vi "Consulta bd v03.vi"(8 "error in (no error)":errorcluster, 11 "Database":T4) -> (0 "error out":errorcluster)   [LabVIEW 2017]
uses:
  <vilib>/addons/database/Connection.llb/Conn ObjectReference.ctl
  <vilib>/GPower/Array/Library/RemDup/RemDup_Str.vi
  <vilib>/GPower/Array/Library/RemDup/RemDup_Var.vi
  <vilib>/NI/AMC/Update Message Routing Info.vi
  <vilib>/NI/AMC/Create Multiple Messages.vi
  <vilib>/NI/AMC/Read Termination Message.vi
  <vilib>/NI/AMC/Create Single Message.vi
  <vilib>/NI/AMC/Send Message.vi
  <vilib>/NI/AMC/Globals.vi
  <userlib>/_OpenG.lib/array/array.llb/Sort 1D Array (String)__ogtk.vi
  <vilib>/addons/database/_DB Variant To Data/Database Variant To Data.xnode
  <vilib>/addons/database/NI_Database_API.lvlib
  <vilib>/NI/AMC/AMC.lvlib
  <vilib>/GPower/Array/GPArray.lvlib
panel:
  in  "System Tab":T1(tab)
  out "Picture":picture
  out "Horas por trabajador":T2(array[cluster])
  out "Horas totales (hh:mm)":string
  out "1D Array":T3(array[cluster])
  in  "Proyectos":string(combo)
  in  "Time Stamp Array":timestamp[](array[timestamp])
  in  "Salir":bool
  in  "Consultar":bool
  in  "Fecha de finalización":timestamp format="%<%.0X %x>T"
  in  "Fecha de inicio":timestamp format="%<%.0X %x>T"
  # "Consulta Base de Datos"
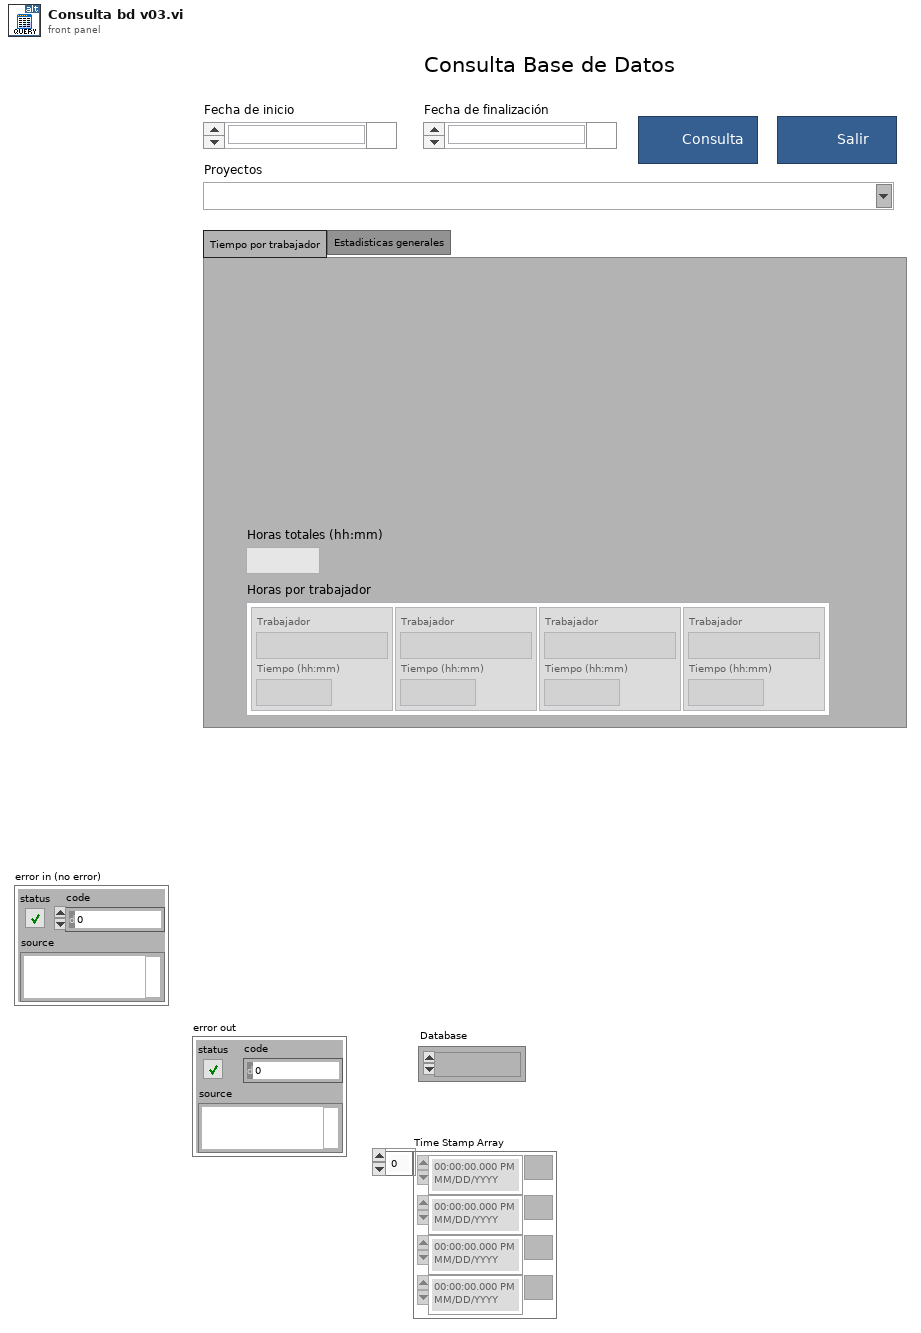
[diagram p1: front panel]
types:
  T1 = enum32{"Tiempo por trabajador", "Estadisticas generales"}
  T2 = cluster{"Trabajador":string, "Tiempo (hh:mm) ":string}[]
  T3 = cluster{"Trabajador":string, "Tarea":string, "Inicio":string, "Fin":string, "Duracion":dbl}[]
  T4 = typedef "NI_Database_API.lvlib/Conn ObjectReference.ctl" = refnum<k1>
  T5 = typedef "AMC.lvlib/Message Queue.ctl" = refnum<queue>
  T6 = cluster{"Trabajador":string, "Tarea":string, "Inicio":string, "Fin":string, "Duracion":i32}[]
  T7 = typedef "LVBoundsTypeDef.ctl" = cluster{"Width":u32, "Height":u32}
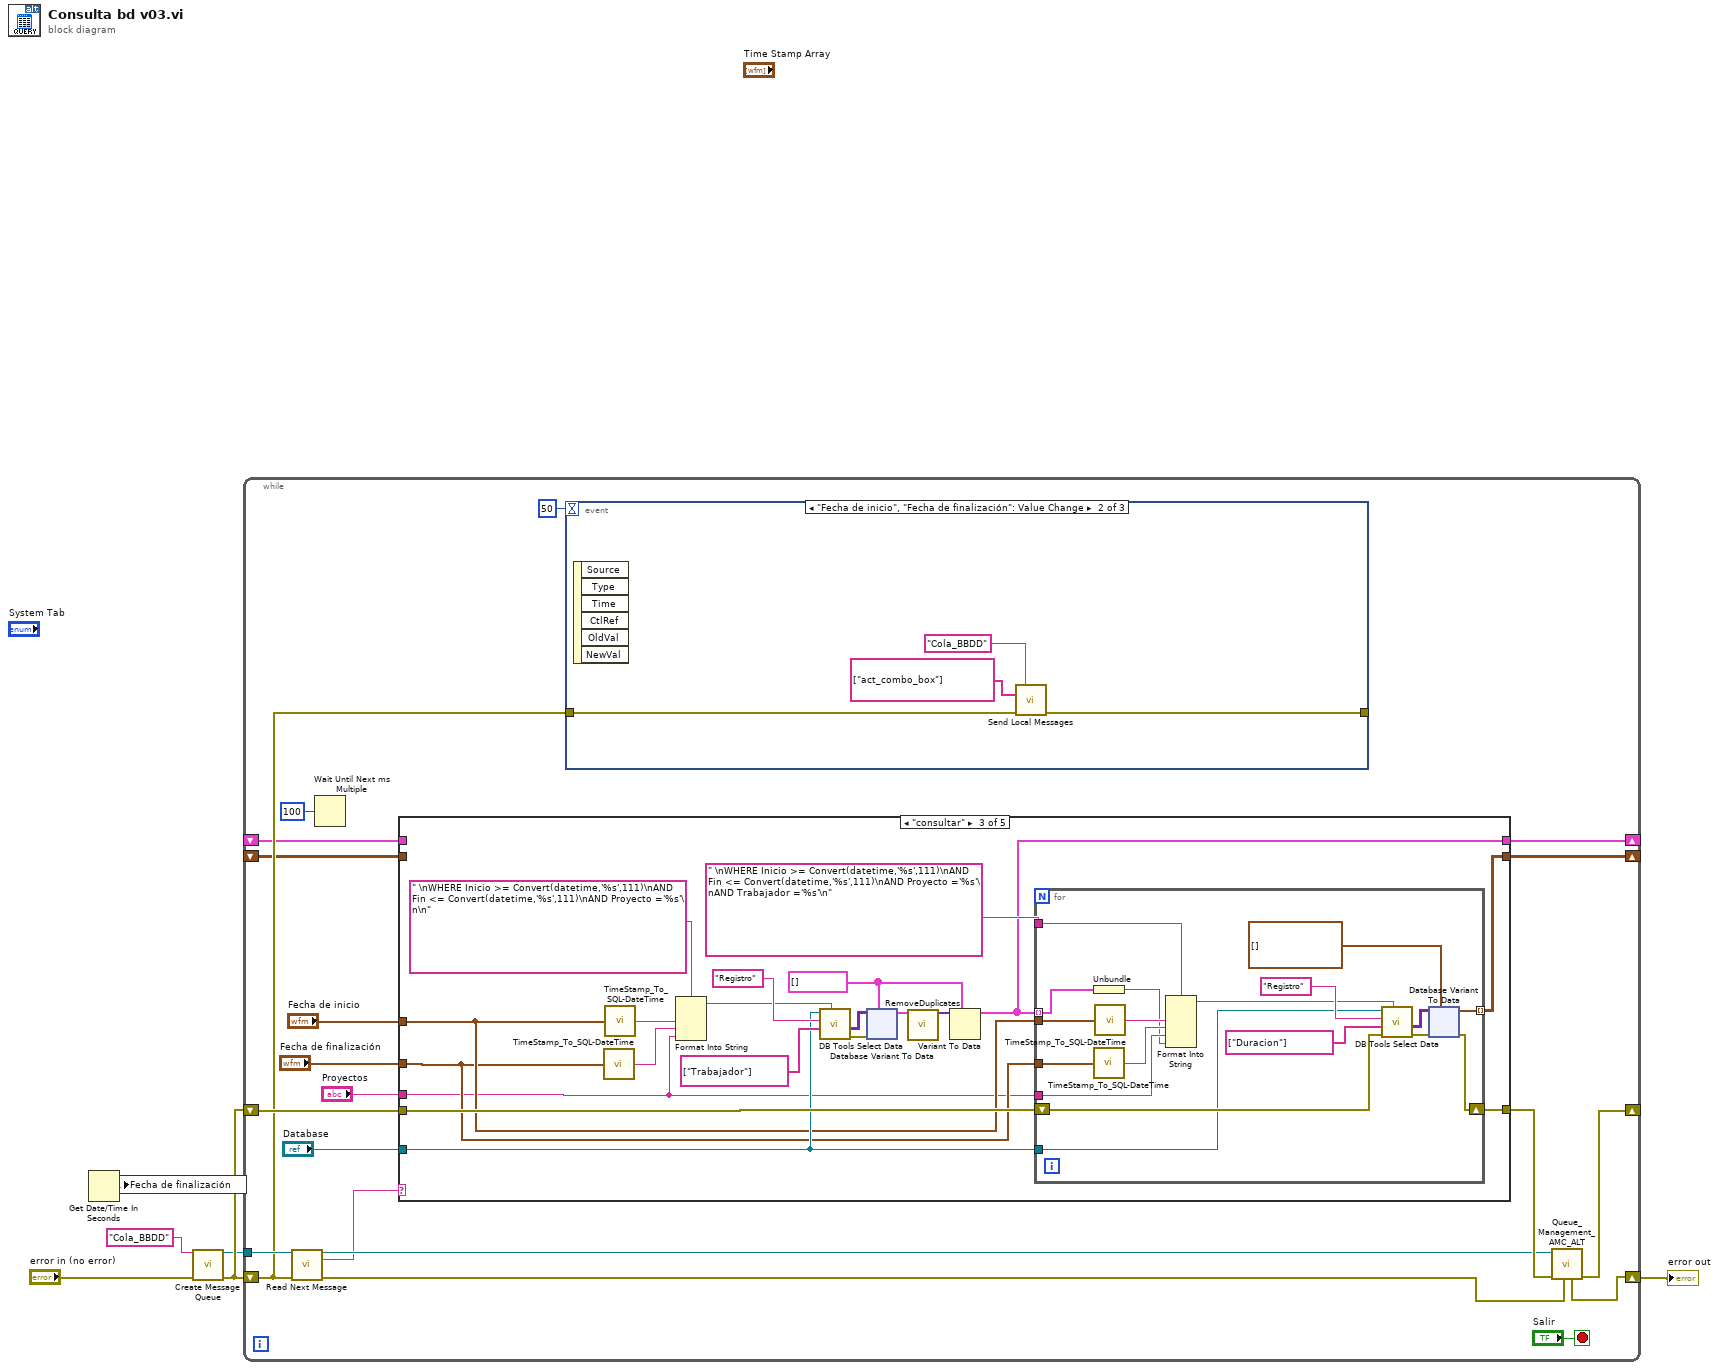
[diagram p0: block diagram]
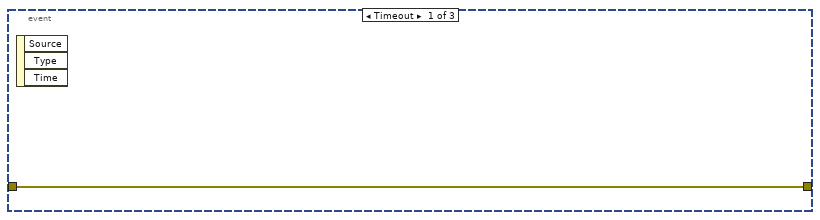
[diagram p2: hidden frame]
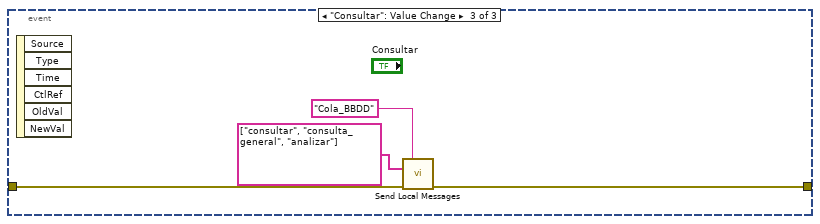
[diagram p3: hidden frame]
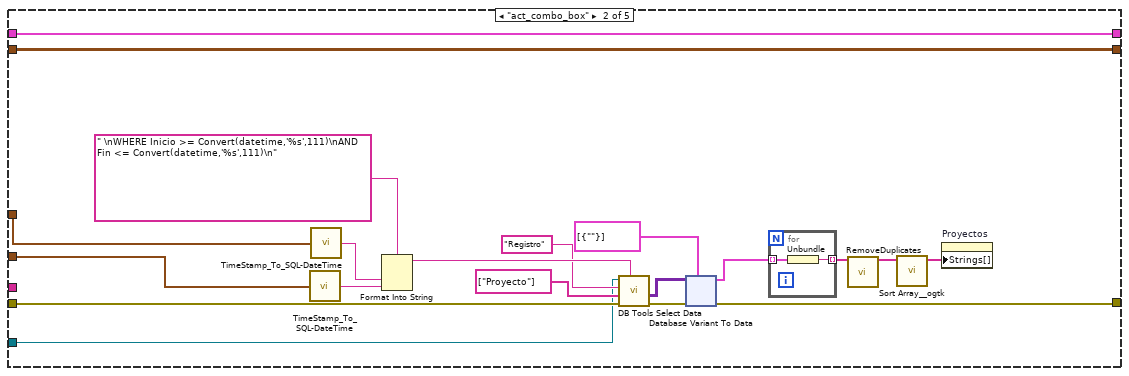
[diagram p5: hidden frame]
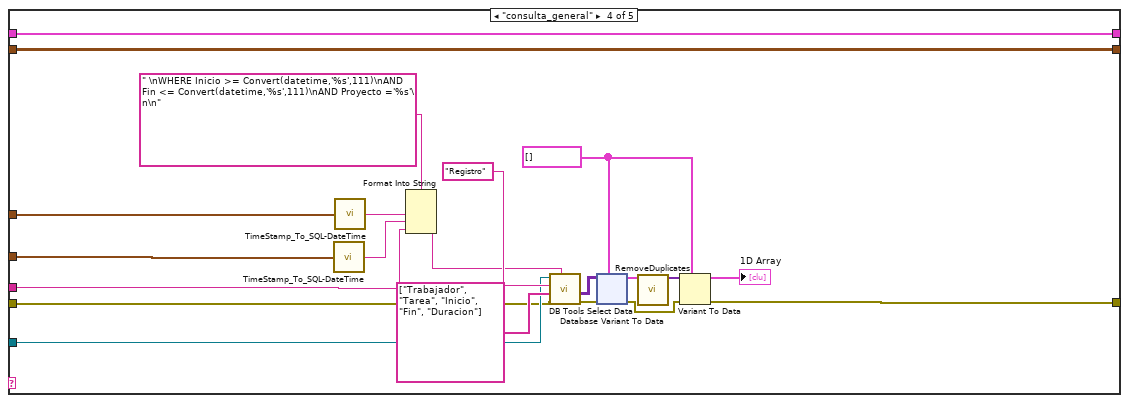
[diagram p6: hidden frame]
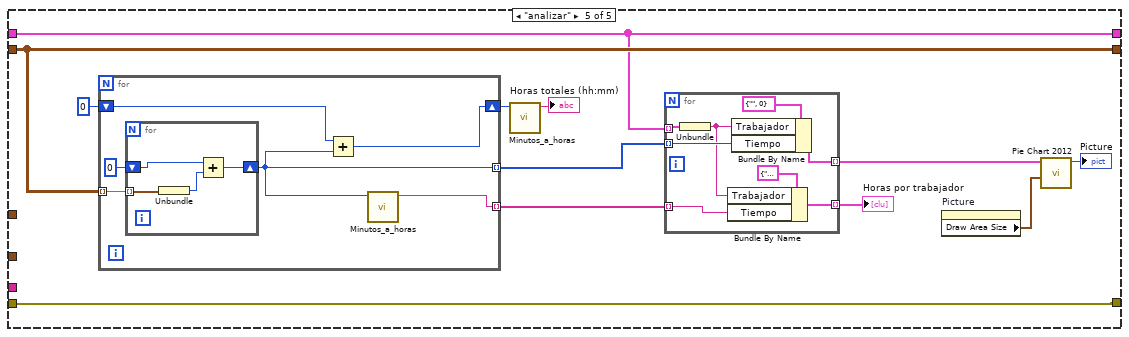
[diagram p7: hidden frame]
diagram:
  n1 = Get Date/Time In Seconds() -> (seconds since 1Jan1904=w3:timestamp)
  n2 = local write "Fecha de finalización"(w3) -> ()
  n3 = call <vilib>:"Create Message Queue.vi"("message queue name"="Cola_BBDD", "error in"="error in (no error)") -> ("message queue out"=w1:T5, "error out"=w2:errorcluster)  [unwired: 12 in]
  n4 = while {
    shift-right: [w18] -> w6
    shift-left: w2 -> [w13]
    tunnel: w1 -> [w20]
    shift-right: [w16] -> _
    shift-left: w2 -> [w21]
    shift-right: [w11] -> _
    shift-left: _ -> [w10]
    shift-right: [w9] -> _
    shift-left: _ -> [w8]
    stop <- "Salir" stop-if-true
    n5 = call <vilib>:"Read Next Message.vi"("message queue in"=w20, "error in"=w13) -> ("message queue out"=w15:T5, "message name"=w14:string, "error out"=w19:errorcluster)  [unwired: 6 in, 5 out]
    n6 = Wait Until Next ms Multiple(millisecond multiple=u32 100) -> ()  [unwired: 1 out]
    n7 = case shown="\"consultar\"" w14 {
      tunnel: w21 -> [w38 w47 w120 w226 w419]
      tunnel: [w38 w44 w121 w224 w419] -> w17
      tunnel: "Fecha de inicio" -> [_ w46 w105 w230 _]
      tunnel: "Fecha de finalización" -> [_ w48 w104 w229 _]
      tunnel: "Database" -> [_ w45 w111 w235 _]
      tunnel: [w37 w43 w116 w227 w416] -> w11
      tunnel: w10 -> [w37 w43 _ w227 w416]
      tunnel: [w36 w42 w103 w223 w414] -> w9
      tunnel: w8 -> [w36 w42 _ w223 w414]
      tunnel: "Proyectos" -> [_ _ w102 w228 _]
      frame "", Default {
      }
      frame "act_combo_box" {
        n8 = call "TimeStamp_To_SQL-DateTime.vi"("time stamp"=w48) -> ("date/time string"=w55:string)
        n9 = call "TimeStamp_To_SQL-DateTime.vi"("time stamp"=w46) -> ("date/time string"=w56:string)
        n10 = Format Into String(format string=" \nWHERE Inicio >= Convert(datetime,'%s',111)\nAND Fin <= Convert(datetime,'%s',111)\n" ("condition"), w56, w55) -> (resulting string=w52:string)  [unwired: 2 in, 1 out]
        n11 = call <vilib>:"DB Tools Select Data.vi"("condition"=w52, "error in (no error)"=w47, "columns"=string[] ["Proyecto"], "table"="Registro", "connection reference"=w45) -> ("error out"=w53:errorcluster, "data"=w58:variant[][])  [unwired: 1 in, 1 out]
        n12 = xnode "Database Variant To Data"("database variant"=w58, "error in (no error)"=w53, "type"=cluster{string}[] [{""}] ("Waveform Graph")) -> ("data"=w50:cluster{string}[], "error out"=w44:errorcluster)
        n13 = for {
          tunnel: w50 -> [w101] mode=indexing
          tunnel: [w100] -> w41 mode=indexing
          n14 = Unbundle(w101) -> (w100:string)
        }
        n15 = call-poly <vilib>:"RemoveDuplicates.vi"("Array"=w41) -> ("Array Without Duplicates"=w40:string[])  [unwired: 12 in, 2 out]
        n16 = call-poly <userlib>:"Sort Array__ogtk.vi"("Array in"=w40) -> ("Sorted Array out"=w39:string[])  [unwired: 9 in, 1 out]
        n17 = property on="Proyectos" class="CmbBox"("Strings[]"=w39) -> ()  [unwired: 2 in, 2 out]
      }
      frame "consultar" {
        w107 = cluster{"Trabajador":string}[] []
        n18 = call "TimeStamp_To_SQL-DateTime.vi"("time stamp"=w104) -> ("date/time string"=w117:string)
        n19 = call "TimeStamp_To_SQL-DateTime.vi"("time stamp"=w105) -> ("date/time string"=w118:string)
        n20 = Format Into String(format string=" \nWHERE Inicio >= Convert(datetime,'%s',111)\nAND Fin <= Convert(datetime,'%s',111)\nAND Proyecto ='%s'\n\n" ("condition"), w118, w117, w102) -> (resulting string=w110:string)  [unwired: 2 in, 1 out]
        n21 = call <vilib>:"DB Tools Select Data.vi"("condition"=w110, "columns"=string[] ["Trabajador"], "table"="Registro", "connection reference"=w111) -> ("error out"=w113:errorcluster, "data"=w112:variant[][])  [unwired: 2 in, 1 out]
        n22 = xnode "Database Variant To Data"("database variant"=w112, "error in (no error)"=w113, "type"=w107) -> ("data"=w109:cluster{"Trabajador":string}[])  [unwired: 1 out]
        n23 = call-poly <vilib>:"RemoveDuplicates.vi"("Array"=w109) -> ("Array with duplicates removed"=w106:variant[])  [unwired: 12 in, 2 out]
        n24 = Variant To Data(type=w107, Variant=w106) -> (data=w103:cluster{"Trabajador":string}[])  [unwired: 1 in, 1 out]
        n25 = for {
          tunnel: [w173] -> w116 mode=indexing
          tunnel: w111 -> [w172]
          tunnel: " \nWHERE Inicio >= Convert(datetime,'%s',111)\nAND Fin <= Convert(datetime,'%s',111)\nAND Proyecto ='%s'\nAND Trabajador ='%s'\n" ("condition") -> [w169]
          tunnel: w102 -> [w168]
          shift-right: [w180] -> w121
          shift-left: w120 -> [w179]
          tunnel: w103 -> [w167] mode=indexing
          tunnel: w105 -> [w164]
          tunnel: w104 -> [w163]
          n26 = Unbundle(w167) -> ("Trabajador"=w166:string)
          n27 = call "TimeStamp_To_SQL-DateTime.vi"("time stamp"=w163) -> ("date/time string"=w171:string)
          n28 = call "TimeStamp_To_SQL-DateTime.vi"("time stamp"=w164) -> ("date/time string"=w170:string)
          n29 = Format Into String(format string=w169, w170, w171, w168, w166) -> (resulting string=w165:string)  [unwired: 2 in, 1 out]
          n30 = call <vilib>:"DB Tools Select Data.vi"("condition"=w165, "error in (no error)"=w179, "columns"=string[] ["Duracion"], "table"="Registro", "connection reference"=w172) -> ("error out"=w177:errorcluster, "data"=w178:variant[][])  [unwired: 1 in, 1 out]
          n31 = xnode "Database Variant To Data"("database variant"=w178, "error in (no error)"=w177, "type"=cluster{"Duracion":i32}[] []) -> ("data"=w173:cluster{"Duracion":i32}[], "error out"=w180:errorcluster)
        }
      }
      frame "consulta_general" {
        w232 = T6 []
        n32 = call "TimeStamp_To_SQL-DateTime.vi"("time stamp"=w229) -> ("date/time string"=w240:string)
        n33 = call "TimeStamp_To_SQL-DateTime.vi"("time stamp"=w230) -> ("date/time string"=w241:string)
        n34 = Format Into String(format string=" \nWHERE Inicio >= Convert(datetime,'%s',111)\nAND Fin <= Convert(datetime,'%s',111)\nAND Proyecto ='%s'\n\n" ("condition"), w241, w240, w228) -> (resulting string=w234:string)  [unwired: 2 in, 1 out]
        n35 = call <vilib>:"DB Tools Select Data.vi"("condition"=w234, "error in (no error)"=w226, "columns"=string[] ["Trabajador", "Tarea", "Inicio", "Fin", "Duracion"], "table"="Registro", "connection reference"=w235) -> ("error out"=w237:errorcluster, "data"=w236:variant[][])  [unwired: 1 in, 1 out]
        n36 = xnode "Database Variant To Data"("database variant"=w236, "error in (no error)"=w237, "type"=w232) -> ("data"=w233:T6, "error out"=w225:errorcluster)
        n37 = call-poly <vilib>:"RemoveDuplicates.vi"("Array"=w233) -> ("Array with duplicates removed"=w231:variant[])  [unwired: 12 in, 2 out]
        n38 = Variant To Data(error in=w225, type=w232, Variant=w231) -> (data=→"1D Array":T6, error out=w224:errorcluster)
      }
      frame "analizar" {
        n39 = for {
          tunnel: w416 -> [w433] mode=indexing
          tunnel: [w430] -> w415 mode=indexing
          tunnel: [w431] -> w412 mode=indexing
          shift-right: [w429] -> w409
          shift-left: 0 -> [w428]
          n40 = for {
            tunnel: w433 -> [w437] mode=indexing
            shift-right: [w434] -> w430
            shift-left: 0 ("Duracion") -> [w436]
            n41 = Unbundle(w437) -> ("Duracion"=w435:i32)
            n42 = Add(x=w436, y=w435) -> (x+y=w434:i32)
          }
          n43 = Add(x=w428, y=w430) -> (x+y=w429:i32)
          n44 = call "Minutos_a_horas.vi"("Duracion"=w430) -> ("String"=w431:string)  [unwired: 10 in]
        }
        n45 = call "Minutos_a_horas.vi"("Duracion"=w409) -> ("String"=→"Horas totales (hh:mm)":string)  [unwired: 10 in]
        n46 = for {
          tunnel: w414 -> [w426] mode=indexing
          tunnel: w415 -> [w425] mode=indexing
          tunnel: [w424] -> w413 mode=indexing
          tunnel: w412 -> [w420] mode=indexing
          tunnel: [w421] -> w411 mode=indexing
          n47 = Unbundle(w426) -> ("Trabajador"=w423:string)
          n48 = Bundle By Name(cluster=cluster{"Trabajador":string, "Tiempo":string} {"Trabajador"="", "Tiempo"=""}, "Trabajador"=w423, "Tiempo"=w420) -> (w421:cluster{"Trabajador":string, "Tiempo":string})
          n49 = Bundle By Name(cluster=cluster{"Trabajador":string, "Tiempo":i32} {"Trabajador"="", "Tiempo"=0}, "Trabajador"=w423, "Tiempo"=w425) -> (w424:cluster{"Trabajador":string, "Tiempo":i32})
        }
        "Horas por trabajador" <- w411
        n50 = property on="Picture" class="Pict"() -> ("Draw Area Size"=w417:T7)  [unwired: 2 in, 2 out]
        n51 = call "Pie Chart 2012.vi"("Draw Area Size"=w417, "Array"=w413) -> ("Picture"=→"Picture":picture)  [unwired: 9 in]
      }
    }
    n52 = event shown="[1] \"Fecha de inicio\", \"Fecha de finalización\": Value Change" {
      selector: _ -> [_ _ _]
      dyn-events: _ -> [_ _ _]
      timeout: 50 -> [_ _ _]
      tunnel: w13 -> [w27 w29 w33]
      tunnel: [w27 w28 w32] -> _
      event Timeout {
        n53 = event-data() -> ()  [unwired: 1 in, 3 out]
      }
      event "Fecha de inicio", "Fecha de finalización": Value Change {
        n54 = event-data() -> ()  [unwired: 1 in, 6 out]
        n55 = call <vilib>:"Send Local Messages.vi"("receiver process (\"\" - local)"="Cola_BBDD" ("receiver process (\"\" - local)"), "message names"=string[] ["act_combo_box"] ("message name"), "error in"=w29) -> ("error out"=w28:errorcluster)  [unwired: 10 in, 2 out]
      }
      event "Consultar": Value Change {
        n56 = event-data() -> ()  [unwired: 1 in, 6 out]
        n57 = call <vilib>:"Send Local Messages.vi"("receiver process (\"\" - local)"="Cola_BBDD" ("receiver process (\"\" - local)"), "message names"=string[] ["consultar", "consulta_general", "analizar"] ("message name"), "error in"=w33) -> ("error out"=w32:errorcluster)  [unwired: 10 in, 2 out]
      }
    }
    n58 = call "Queue_Management_AMC_ALT.vi"("queue error in"=w19, "system error in"=w17, "message queue in"=w15) -> ("system error out"=w16:errorcluster, "queue error out"=w18:errorcluster)  [unwired: 5 in, 2 out]
  }
  "error out" <- w6
